vi "CS-4 Get Units.vi"(0 "VISA session":refnum<visa-resource-name>, 1 "error in (no error)":errorcluster) -> (2 "dup VISA session":refnum<visa-resource-name>, 3 "response out":string, 4 "units":enum16{"Amps", "Kilogauss", "Tesla"}(ring)=enum."Kilogauss", 5 "error out":errorcluster)   [LabVIEW 2016]
doc: "CS-4 Get Units.vi will return the units both as a string and as an enumerated type."
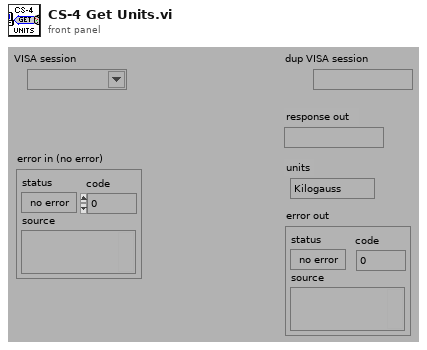
[diagram p1: front panel]
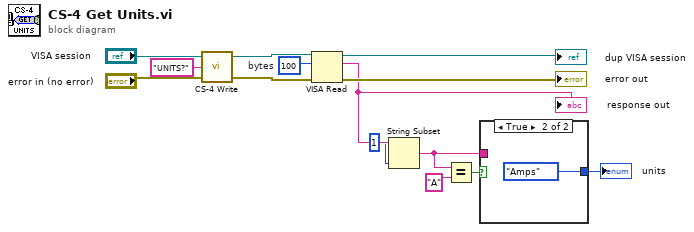
[diagram p0: block diagram]
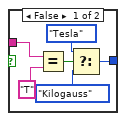
[diagram p2: hidden frame]
diagram:
  w8 = u32 100  # bytes
  n1 = call "CS-4 Write.vi"("error in (no error)"="error in (no error)", "write buffer (\"\")"="UNITS?", "VISA session"="VISA session") -> ("error out"=w11:errorcluster, "dup VISA session"=w12:refnum<visa-resource-name>)  [unwired: 1 out]
  n2 = VISA Read(VISA resource name=w12, byte count=w8, error in (no error)=w11) -> (VISA resource name out=→"dup VISA session":refnum<visa-resource-name>, read buffer=w6:string, error out=→"error out":errorcluster)  [unwired: 1 out]
  "response out" <- w6
  n3 = String Subset(string=w6, length (rest)=1 ("length")) -> (substring=w2:string)  [unwired: 1 in]
  n4 = Equal?(x=w2, y="A") -> (x = y?=w1:bool)
  n5 = case shown="True" w1 {
    tunnel: [w20 enum16{"Amps", "Kilogauss", "Tesla"}."Amps" ("units")] -> w3
    tunnel: w2 -> [w19 _]
    frame False {
      n6 = Equal?(x=w19, y="T") -> (x = y?=w17:bool)
      n7 = Select(t=enum16{"Amps", "Kilogauss", "Tesla"}."Tesla" ("Units"), s=w17, f=enum16{"Amps", "Kilogauss", "Tesla"}."Kilogauss" ("units")) -> (s? t:f=w20:enum16{"Amps", "Kilogauss", "Tesla"})
    }
    frame True {
    }
  }
  "units" <- w3
